vi "4110_Volt _Chan Config Dialog.vi"(8 "error in (no error)":errorcluster, 11 "Data Entry Limits:Maximum":dbl) -> (0 "error out":errorcluster, 1 "sense (out)":T1=1008 items=["Local"=1008, "Remote"=1009], 2 "Current Limit (out)":dbl, 3 "Initial Voltage Value (out)":dbl, 4 "Cancel (out)":bool, 5 "Number of Voltage Output Channels to Add? (out)":i16)   [LabVIEW 2018]
uses:
  <instrlib>/niDCPower/nidcpower.llb/niDCPower Sense.ctl
panel:
  in  "Cancel":bool
  in  "OK Button":bool
  in  "Current Limit":dbl format="%.4f"
  in  "Initial Voltage Value":dbl
  in  "sense":T1=1008 caption="Sense" items=["Local"=1008, "Remote"=1009]
  in  "Number of Voltage Output Channels to Add?":i16
  # "Voltage Channels"
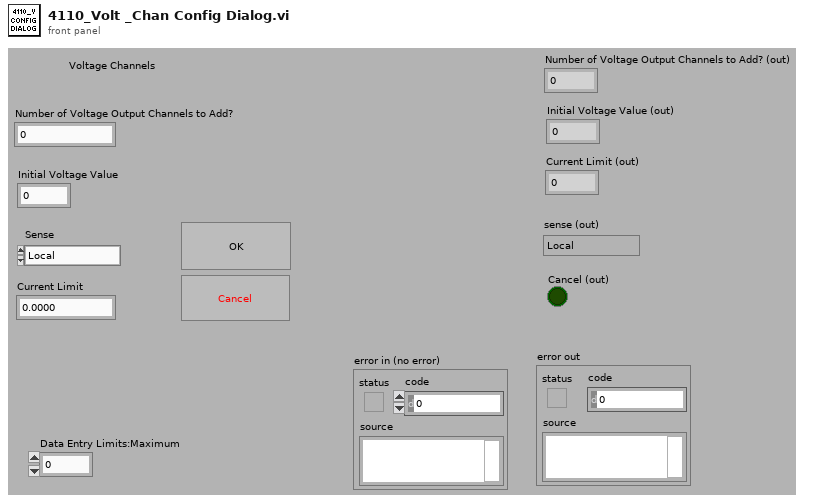
[diagram p1: front panel]
types:
  T1 = typedef "niDCPower Sense.ctl" = i32
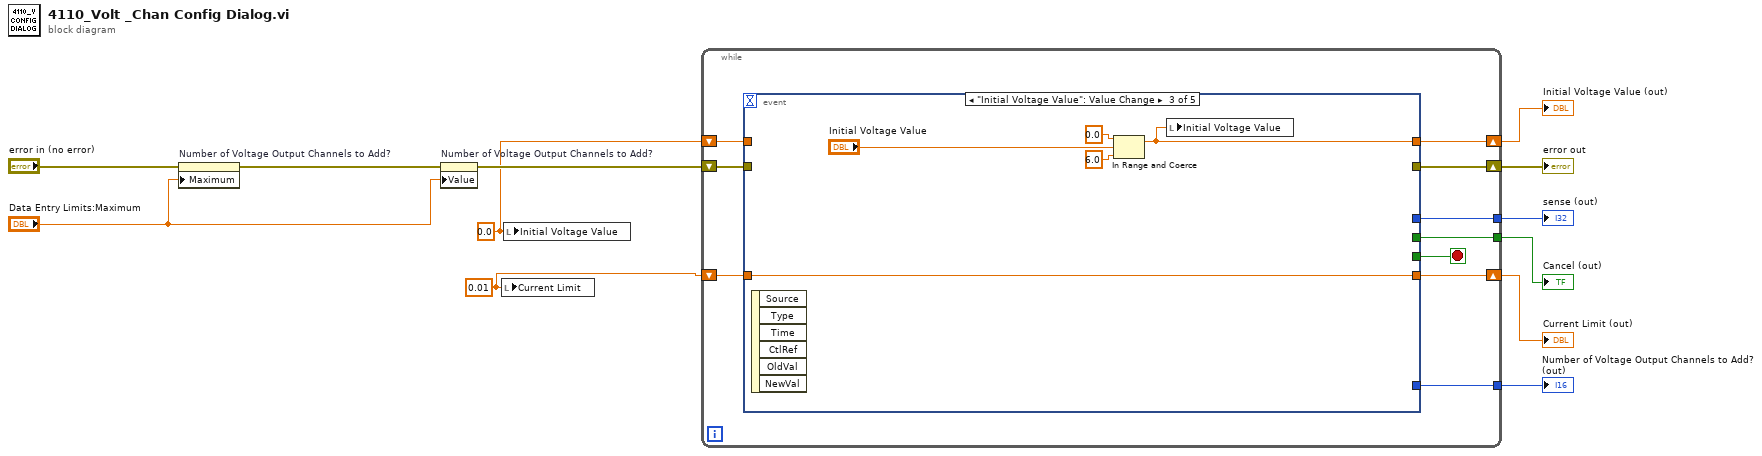
[diagram p0: block diagram]
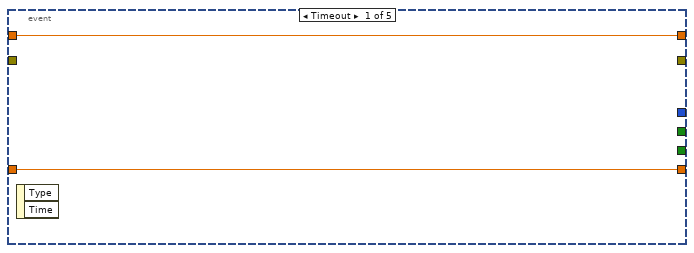
[diagram p2: hidden frame]
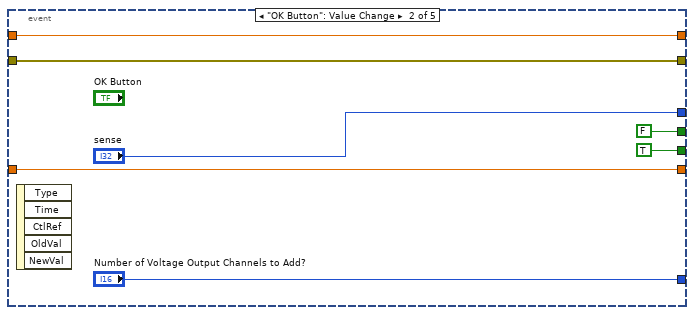
[diagram p3: hidden frame]
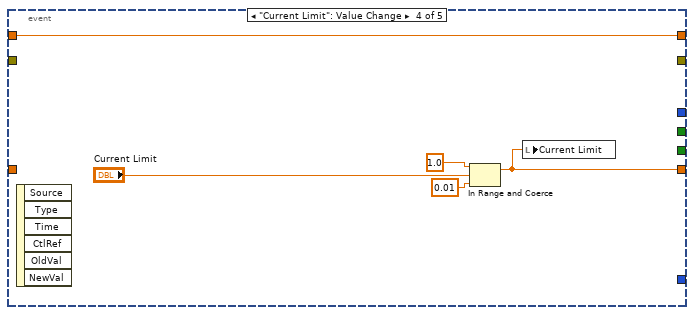
[diagram p4: hidden frame]
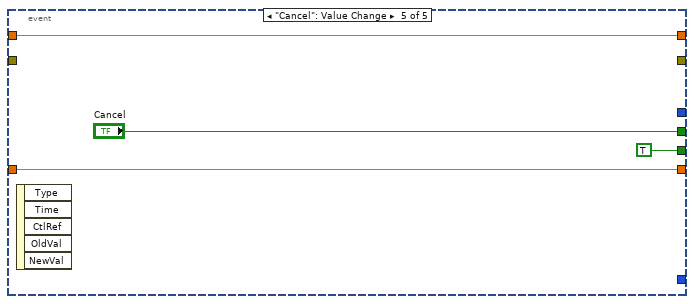
[diagram p5: hidden frame]
diagram:
  w1 = 0.0 ("Initial Voltage Value")
  w2 = 0.01 ("Current Limit")
  n1 = property on="Number of Voltage Output Channels to Add?" class="DigNum (strict)"(error in="error in (no error)", "Maximum"="Data Entry Limits:Maximum") -> (error out=w12:errorcluster)  [unwired: 1 in, 1 out]
  n2 = property on="Number of Voltage Output Channels to Add?" class="DigNum (strict)"(error in=w12, "Value"="Data Entry Limits:Maximum") -> (error out=w10:errorcluster)  [unwired: 1 in, 1 out]
  n3 = local write "Current Limit"(w2) -> ()
  n4 = local write "Initial Voltage Value"(w1) -> ()
  n5 = while {
    tunnel: [w19] -> w7
    tunnel: [w17] -> w5
    tunnel: [w16] -> w3
    shift-right: [w21] -> w9
    shift-left: w10 -> [w22]
    shift-right: [w20] -> w8
    shift-left: w2 -> [w14]
    shift-right: [w18] -> w6
    shift-left: w1 -> [w13]
    stop <- w15 stop-if-true
    n6 = event shown="[2] \"Initial Voltage Value\": Value Change" {
      selector: _ -> [_ _ _ _ _]
      dyn-events: _ -> [_ _ _ _ _]
      timeout: _ -> [_ _ _ _ _]
      tunnel: [w24 w26 w36 w38 w43] -> w20
      tunnel: [_ "sense" _ _ _] -> w19
      tunnel: [w23 w25 w32 w37 w42] -> w18
      tunnel: w22 -> [_ w30 _ _ _]
      tunnel: [_ w30 _ _ _] -> w21
      tunnel: [_ FALSE ("Cancel") _ _ "Cancel"] -> w17
      tunnel: [_ "Number of Voltage Output Channels to Add?" _ _ _] -> w16
      tunnel: [_ TRUE ("Cancel") _ _ TRUE ("Cancel")] -> w15
      tunnel: w14 -> [w24 w26 w36 _ w43]
      tunnel: w13 -> [w23 w25 _ w37 w42]
      event Timeout {
        n7 = event-data() -> ()  [unwired: 1 in, 2 out]
      }
      event "OK Button": Value Change {
        n8 = event-data() -> ()  [unwired: 1 in, 5 out]
      }
      event "Initial Voltage Value": Value Change {
        n9 = event-data() -> ()  [unwired: 1 in, 6 out]
        n10 = In Range and Coerce(upper limit=0.0, x="Initial Voltage Value", lower limit=6.0) -> (coerced(x)=w32:dbl)  [unwired: 1 out]
        n11 = local write "Initial Voltage Value"(w32) -> ()
      }
      event "Current Limit": Value Change {
        n12 = event-data() -> ()  [unwired: 1 in, 6 out]
        n13 = In Range and Coerce(upper limit=1.0, x="Current Limit", lower limit=0.01) -> (coerced(x)=w38:dbl)  [unwired: 1 out]
        n14 = local write "Current Limit"(w38) -> ()
      }
      event "Cancel": Value Change {
        n15 = event-data() -> ()  [unwired: 1 in, 5 out]
      }
    }
  }
  "error out" <- w9
  "Current Limit (out)" <- w8
  "sense (out)" <- w7
  "Initial Voltage Value (out)" <- w6
  "Cancel (out)" <- w5
  "Number of Voltage Output Channels to Add? (out)" <- w3
